vi "LVDimInterface.dim_set_occurrence_ref.vi"(2 "occurrence":refnum<k4>, 5 "error in (no error)":errorcluster) -> (19 "error out":errorcluster)   [LabVIEW 2016, in "LVDimInterface.lvlib"]
doc: "This routine can be called by a server or a client program before receiving DIM services to register the reference of an occurrence to the dimWrapper shared library. The library will fire (set) the occurrence when new service data is available.\n\n\n\nHistory: 24-OCT-2007, Dietrich Beck\n\nCopyright (C)\nGesellschaft für Schwerionenforschung, GSI\nPlanckstr. 1\n64291 Darmstadt\nGermany\n\nContact: D.Beck@gsi.de \n\nThis program is free software; you can redistribute it and/or modify it under the terms of the \nGNU General Public License as published by the Free Software Foundation; either version 2 of the license, or (at your option) any later version.\n\nThis program is distributed in the hope that it will be useful, but WITHOUT ANY WARRANTY; without even the implied warranty of MERCHANTABILITY or FITNESS FOR A PARTICULAR PURPOSE. See the GNU General License for more details (http://www.gnu.org).\n\nGesellschaft für Schwerionenforschung, GSI\nPlanckstr. 1, 64291 Darmstadt, Germany\nFor all questions and ideas contact D. Beck.\nLast update: 16-DEC-2005"
uses:
  LVDimInterface.lvlib
  bin/libDimWrapper.dll
  bin/libDimWrapper.so
  bin/libDimWrapperSPL.dll
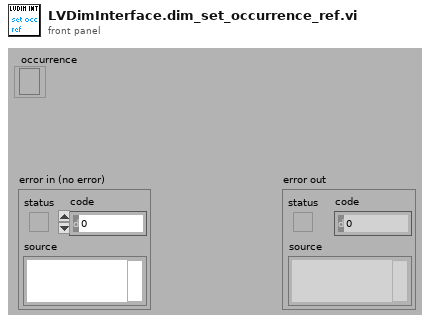
[diagram p1: front panel]
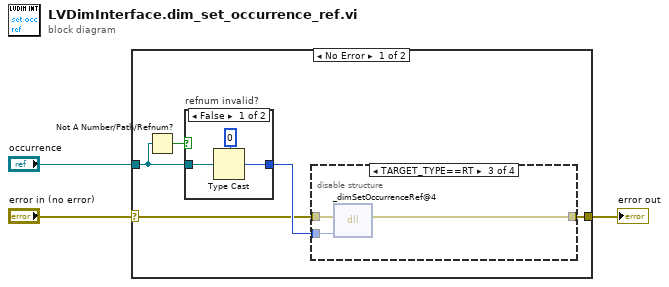
[diagram p0: block diagram]
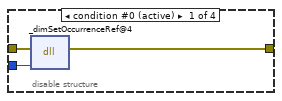
[diagram p2: hidden frame]
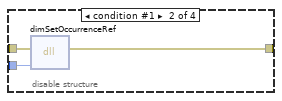
[diagram p3: hidden frame]
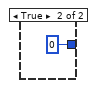
[diagram p5: hidden frame]
diagram:
  n1 = case shown="No Error" "error in (no error)" {
    selector: "error in (no error)" -> [w5 w23]
    tunnel: "occurrence" -> [w6 _]
    tunnel: [w4 w23] -> w3
    frame No Error {
      n2 = Not A Number/Path/Refnum?(number/path/refnum=w6) -> (NaN/Path/Refnum?=w7:bool)
      n3 = case "refnum invalid?" shown="False" w7 {
        tunnel: w6 -> [w21 _]
        tunnel: [w20 u32 0] -> w8
        frame False {
          n4 = Type Cast(type=u32 0, x=w21) -> (*(type *) &x=w20:u32)
        }
        frame True {
        }
      }
      n5 = disable-structure "Conditional Disable Structure" shown="TARGET_TYPE==RT" {
        disable-tunnel: w8 -> [w11 w14 w17 _]
        disable-tunnel: w5 -> [w10 w13 w16 w18]
        disable-tunnel: [w9 w12 w15 w18] -> w4
        frame condition #0 (active) {
          n6 = dll-call lib="D:/Git/DimLVEvent/bin/libDimWrapper.dll" fn="_dimSetOccurrenceRef@4"(error in=w10, "occurrenceRef"=w11) -> (error out=w9:errorcluster)  [unwired: 4 in, 1 out]
        }
        frame condition #1 {
          n7 = dll-call lib="D:/Git/CSPP/Packages/DimLVEvent/bin/libDimWrapper.so" fn="dimSetOccurrenceRef" label="libDimWrapper.dll:_dimSetOccurrenceRef@4"(error in=w13, "occurrenceRef"=w14) -> (error out=w12:errorcluster)  [unwired: 4 in, 1 out]
        }
        frame condition #2 {
          n8 = dll-call lib="D:/Git/DimLVEvent/bin/libDimWrapperSPL.dll" fn="_dimSetOccurrenceRef@4"(error in=w16, "occurrenceRef"=w17) -> (error out=w15:errorcluster)  [unwired: 4 in, 1 out]
        }
        frame condition #3 {
        }
      }
    }
    frame Error {
    }
  }
  "error out" <- w3
